vi "Add CPU Channels.vi"(8 "error in (no error)":errorcluster, 10 "Number of CPU Cores in":u64, 11 "Item Ref in":T1 format="%.0x") -> (0 "error out":errorcluster, 3 "Item Ref out":T1 format="%.0x")   [LabVIEW 2027, in "System Monitor System Explorer.lvlib"]
uses:
  System Monitor System Explorer.lvlib
  <vilib>/NI VeriStand/Custom Device API/Custom Device Item Ref.ctl
  <vilib>/NI VeriStand/Custom Device API/Custom Device Channel.ctl
  <vilib>/NI VeriStand/Custom Device API/Custom Device Channel Type.ctl
  <vilib>/NI VeriStand/Custom Device API/Custom Device API.lvlib
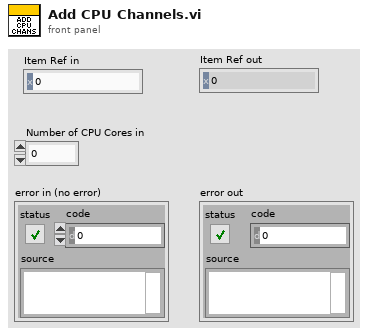
[diagram p1: front panel]
types:
  T1 = typedef "Custom Device API.lvlib/Custom Device Item Ref.ctl" = u64
  T2 = typedef "Custom Device API.lvlib/Custom Device Channel.ctl" = cluster{"Type":T3, "Units":string, "Default Value":dbl, "Faultable":bool, "Scalable":bool}
  T3 = typedef "Custom Device API.lvlib/Custom Device Channel Type.ctl" = enum16{"Input", "Output"}
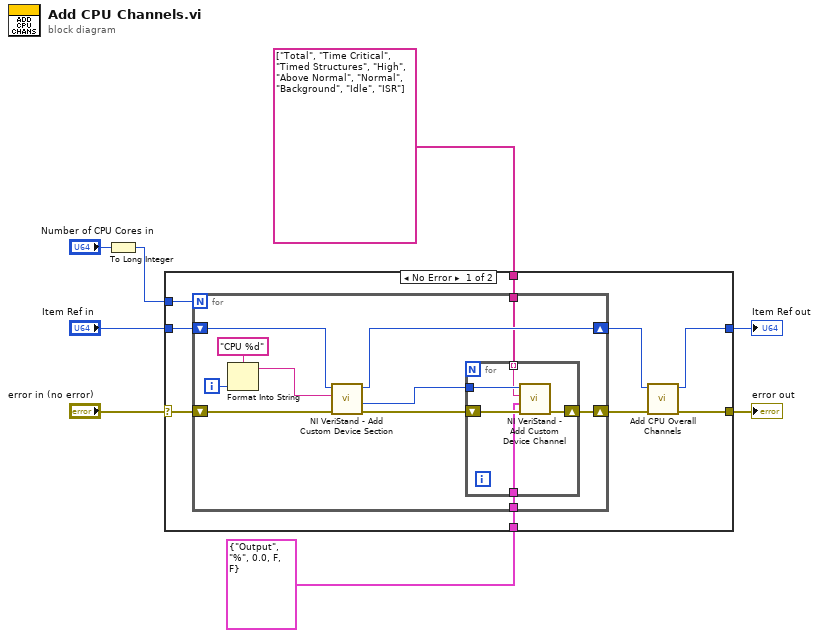
[diagram p0: block diagram]
diagram:
  n1 = To Long Integer(number="Number of CPU Cores in") -> (32bit integer=w1:i32)
  n2 = case shown="No Error" "error in (no error)" {
    selector: "error in (no error)" -> [w13 w34]
    tunnel: w1 -> [w17 _]
    tunnel: [w11 w34] -> w7
    tunnel: [w9 w35] -> w6
    tunnel: "Item Ref in" -> [w16 w35]
    tunnel: T2 {"Type"=enum."Output", "Units"="%", "Default Value"=0.0, "Faultable"=FALSE, "Scalable"=FALSE} ("Channel") -> [w15 _]
    tunnel: string[] ["Total", "Time Critical", "Timed Structures", "High", "Above Normal", "Normal", "Background", "Idle", "ISR"] -> [w14 _]
    frame No Error {
      n3 = for {
        N: w17 -> [_]
        shift-right: [w26] -> w10
        shift-left: w16 -> [w28]
        shift-right: [w20] -> w12
        shift-left: w13 -> [w22]
        tunnel: w15 -> [w19]
        tunnel: w14 -> [w18]
        i -> [w24]
        n4 = Format Into String(format string="CPU %d" ("Section Name"), w24) -> (resulting string=w23:string)  [unwired: 2 in, 1 out]
        n5 = call <vilib>:"NI VeriStand - Add Custom Device Section.vi"("error in (no error)"=w22, "Section Name"=w23, "Parent Ref in"=w28) -> ("error out"=w21:errorcluster, "Section Ptr"=w27:T1, "Parent Ref out"=w26:T1)  [unwired: 5 in, 1 out]
        n6 = for {
          tunnel: w27 -> [w33]
          shift-right: [w31] -> w20
          shift-left: w21 -> [w32]
          tunnel: w19 -> [w30]
          tunnel: w18 -> [w29] mode=indexing
          n7 = call <vilib>:"NI VeriStand - Add Custom Device Channel.vi"("error in (no error)"=w32, "Channel"=w30, "Channel Name"=w29, "Parent Ref in"=w33) -> ("error out"=w31:errorcluster)  [unwired: 4 in, 3 out]
        }
      }
      n8 = call "Add CPU Overall Channels.vi"("error in"=w12, "custom device"=w10) -> ("error out"=w11:errorcluster, "custom device out"=w9:T1)  [unwired: 8 in]
    }
    frame Error {
    }
  }
  "error out" <- w7
  "Item Ref out" <- w6
